vi "SetParam.vi"(8 "error in (no error)":errorcluster caption="entrée d'erreur (pas d'erreur)", 10 "linear_kernel":cluster{"dense_output":bool}={"dense_output"=TRUE}, 11 "Linear_kernel.lvclass":refnum<class "Linear_kernel.lvclass">) -> (0 "error out":errorcluster caption="sortie d'erreur", 3 "Linear_kernel.lvclass":refnum<class "Linear_kernel.lvclass">)   [LabVIEW 2020, in "Linear_kernel.lvclass"]
doc: "Set Parameters"
uses:
  Linear_kernel.lvclass
  Linear_kernel.lvclass/Linear_kernel.ctl
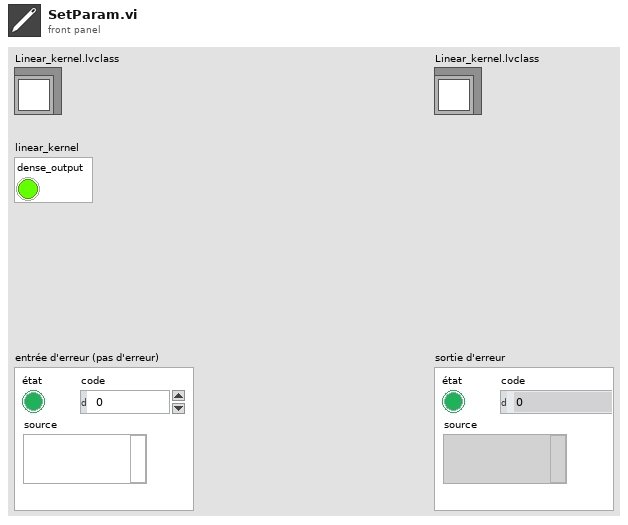
[diagram p1: front panel]
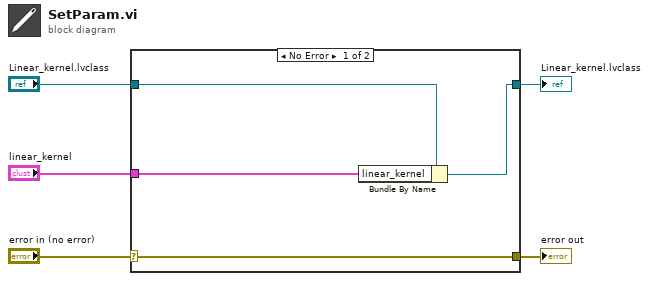
[diagram p0: block diagram]
diagram:
  n1 = case shown="No Error" "error in (no error)" {
    selector: "error in (no error)" -> [w9 w10]
    tunnel: [w9 w10] -> w4
    tunnel: [w7 w11] -> w2
    tunnel: "Linear_kernel.lvclass" -> [w8 w11]
    tunnel: "linear_kernel" -> [w6 _]
    frame No Error {
      n2 = Bundle By Name(cluster=w8, "linear_kernel"=w6) -> (w7:refnum<class "Linear_kernel.lvclass">)
    }
    frame Error {
    }
  }
  "error out" <- w4
  "Linear_kernel.lvclass" <- w2
